vi "RT Main2.vi"() -> ()   [LabVIEW 2019]
uses:
  <vilib>/Platform/TimedLoop/XDataNode/timing_clust.ctl
  <vilib>/Platform/TimedLoop/XDataNode/nitl_modes.ctl
  <vilib>/Platform/TimedLoop/XDataNode/wakeup.ctl
  <vilib>/myRIO/Instrument Drivers/Onboard IO/AI/typedefs/AI Reference.ctl
  <vilib>/myRIO/Common/Instrument Driver Framework/Utilities/typedefs/myRIO Generic Hardware Reference.ctl
  <vilib>/myRIO/Common/Instrument Driver Framework/Utilities/typedefs/Hardware Version Enum.ctl
  <vilib>/myRIO/Common/Instrument Driver Framework/Utilities/typedefs/myRIO v1.0 Reference.ctl
  <vilib>/myRIO/Common/Instrument Driver Framework/Utilities/typedefs/Generic FPGA Reference.ctl
  <vilib>/myRIO/Common/Instrument Driver Framework/myRIO v1.0/AI/typedefs/AI Channels List.ctl
  <vilib>/myRIO/Common/Instrument Driver Framework/myRIO v1.0/AI/typedefs/AI Channels Enum.ctl
  <vilib>/myRIO/Common/Instrument Driver Framework/Utilities/typedefs/Analog Scaling Constants List.ctl
  <vilib>/myRIO/Common/Instrument Driver Framework/Utilities/typedefs/Analog Scaling Constants.ctl
  <vilib>/userDefined/High Color/nirio_resource_hc.ctl
  <vilib>/Simulation/Shared/_Datatypes/SIM SISO Transfer Function.ctl
  <vilib>/myRIO/Instrument Drivers/Onboard IO/AO/typedefs/AO Reference.ctl
  <vilib>/myRIO/Common/Instrument Driver Framework/myRIO v1.0/AO/typedefs/AO Channels List.ctl
  <vilib>/myRIO/Common/Instrument Driver Framework/myRIO v1.0/AO/typedefs/AO Channels Enum.ctl
  <vilib>/Analysis/Matrix/Datatypes/RealMatrix.ctl
  <vilib>/myRIO/Common/Instrument Driver Framework/Utilities/vis/Is FPGA Ref Available.vi
  <vilib>/myRIO/Common/Instrument Driver Framework/myRIO v1.0/AI/vis/myRIO v1.1 Open AI.vi
  <vilib>/myRIO/Instrument Drivers/Onboard IO/AI/vis/Read.vi
  <vilib>/Simulation/DiscreteLinear/Implementation/NILVSim Discrete Transfer Function Direct.llb/SIM Discrete Transfer Function Diagram (SISO).vi
  <vilib>/myRIO/Common/Instrument Driver Framework/myRIO v1.0/AO/vis/myRIO v1.1 Open AO.vi
  <vilib>/myRIO/Instrument Drivers/Onboard IO/AO/vis/Write.vi
  <vilib>/Analysis/7linalg.llb/Real Transpose Matrix.vi
  <vilib>/Analysis/baseanly.llb/Real A x B.vi
  <vilib>/myRIO/Common/Instrument Driver Framework/Utilities/vis/Validate Channels.vi
  <vilib>/myRIO/Common/Instrument Driver Framework/myRIO v1.0/AI/vis/myRIO v1.0 Reserve AI.vi
  <vilib>/Simulation/ContinuousLinear/Implementation/Shared/SIM Transfer Function Support.llb/SIM TransferFunction Normalize to Buffer.vi
  <vilib>/Simulation/DiscreteLinear/Implementation/Shared/SIM Init Discrete States.vi
  <vilib>/Simulation/DiscreteLinear/Implementation/NILVSim Discrete Transfer Function Direct.llb/SIM Transfer Function Direct core (SISO).vi
  <vilib>/myRIO/Common/Instrument Driver Framework/myRIO v1.0/AO/vis/myRIO v1.0 Reserve AO.vi
  <vilib>/myRIO/Common/Instrument Driver Framework/myRIO v1.0/AI/vis/myRIO v1.0 Build MUX Configuration AI.vi
  <vilib>/myRIO/Common/Instrument Driver Framework/myRIO v1.0/Resource Manager/vis/myRIO v1.0 Reserve Channel List.vi
  <vilib>/Simulation/ContinuousLinear/Implementation/Shared/SIM Transfer Function Support.llb/SIM TransferFunction Normalize.vi
  <vilib>/myRIO/Common/Instrument Driver Framework/myRIO v1.0/AO/vis/myRIO v1.0 Build MUX Configuration AO.vi
  <vilib>/myRIO/Common/Instrument Driver Framework/myRIO v1.0/Resource Manager/vis/myRIO v1.0 Reserve Channel.vi
  <vilib>/myRIO/Common/Instrument Driver Framework/myRIO v1.0/Resource Manager/vis/myRIO v1.0 Unreserve Channel.vi
  <vilib>/Simulation/Implementation/Shared/SIM Polynomials.llb/SIM Remove Zero Coefficients (DBL).vi
  <vilib>/myRIO/Common/Instrument Driver Framework/myRIO v1.0/Resource Manager/vis/myRIO v1.0 Build Mutex Name.vi
  <vilib>/Utility/VariantDataType/GetNumericInfo.vi
  <vilib>/Utility/error.llb/Error Cluster From Error Code.vi
  <vilib>/myRIO/Common/Instrument Driver Framework/myRIO v1.0/myRIO v1.1 Open.vi
  <vilib>/myRIO/Common/Instrument Driver Framework/myRIO v1.0/AI/vis/myRIO v1.0 Get Scaling Constants AI.vi
  <vilib>/myRIO/Common/Instrument Driver Framework/Utilities/vis/IO Manager.vi
  <vilib>/myRIO/Common/Instrument Driver Framework/Utilities/vis/Configuration Manager.vi
  <vilib>/myRIO/Common/Instrument Driver Framework/myRIO v1.0/myRIO v1.0 Close.vi
  <vilib>/myRIO/Common/Instrument Driver Framework/myRIO v1.0/AI/vis/myRIO v1.0 Read AI.vi
  <vilib>/Simulation/Implementation/Shared/SIM Polynomials.llb/SIM Divide Polynomials (DBL).vi
  <vilib>/Simulation/Implementation/Shared/SIM BuildSimErr.vi
  <vilib>/myRIO/Common/Instrument Driver Framework/myRIO v1.0/AO/vis/myRIO v1.0 Get Scaling Constants AO.vi
  <vilib>/myRIO/Common/Instrument Driver Framework/myRIO v1.0/AO/vis/myRIO v1.0 Write AO.vi
  <vilib>/Analysis/Matrix/Numeric/Conversions/Array To Matrix - RA.vi
  <vilib>/Analysis/Matrix/Numeric/Multiply/Multiply - R,RM.vi
  <vilib>/platform/TimedLoop/XDataNode/XDataNode.xnode
  <vilib>/myRIO/Express VI/Onboard IO/AI/AI Express VI.xnode
  <vilib>/myRIO/Instrument Drivers/Onboard IO/AI/vis/myRIO AI Open.xnode
  <vilib>/Simulation/Implementation/XNodeFramework/SimXNode/SimX.xnode
  <vilib>/myRIO/Express VI/Onboard IO/AO/AO Express VI.xnode
  <vilib>/myRIO/Instrument Drivers/Onboard IO/AO/vis/myRIO AO Open.xnode
  <vilib>/Platform/TimedLoop/XDataNode/XDNodeRunTimeDep.lvlib
  <vilib>/myRIO/Instrument Drivers/Onboard IO/AI/AI.lvlib
  <vilib>/myRIO/Instrument Drivers/Onboard IO/AO/AO.lvlib
  <vilib>/Analysis/Matrix/NI_Matrix.lvlib
  <vilib>/gmath/NI_Gmath.lvlib
  <vilib>/Analysis/NI_AALPro.lvlib
  <vilib>/Analysis/NI_AALBase.lvlib
panel:
  out "Control Law":string
  in  "Stop EM MLC":bool=TRUE
  out "x[um] 2":dbl(graph)
  out "u[A] 2":dbl(graph)
  out "iteration duration 2":i64(graph)
  in  "max J":dbl
  out "t MLC":dbl
  in  "MLC run time[s]":dbl
  out "J":dbl
  out "Wait For b":bool
  out "State":i16
  in  "PD run time[s]":dbl
  out "t [PD]":dbl
  in  "stop":bool
  in  "Kd":dbl
  in  "Kp":dbl
  out "iteration duration":i64(graph)
  out "u[A]":dbl(graph)
  out "x[um]":dbl(graph)
  in  "Stop EM PD":bool=TRUE
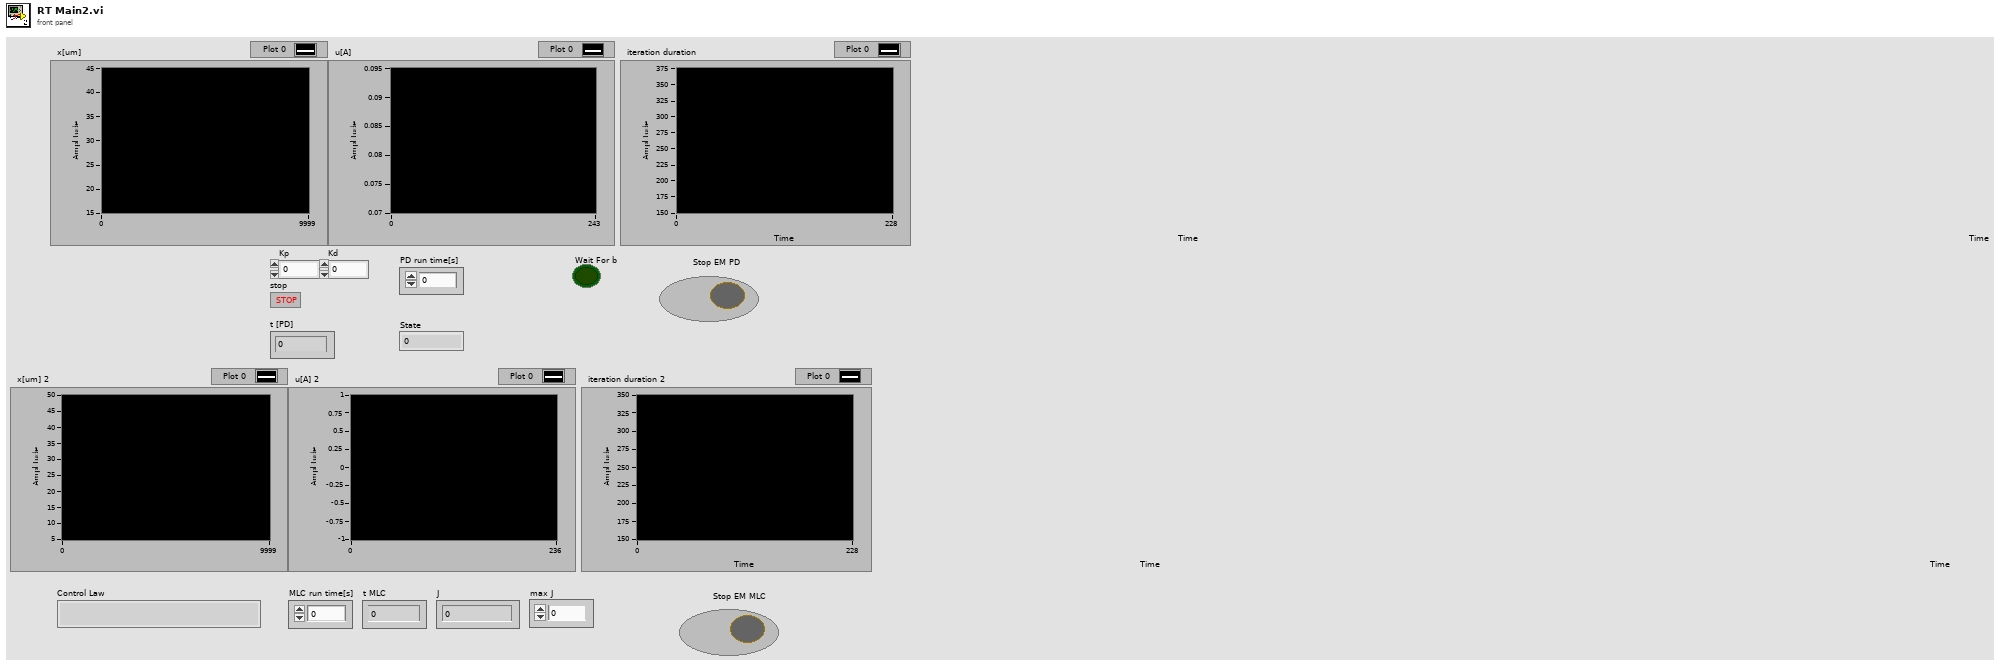
[diagram p1: front panel]
types:
  T1 = typedef "SIM SISO Transfer Function.ctl" = cluster{"Numerator":dbl[], "Denominator":dbl[]}
  T2 = typedef "AO.lvlib/AO Reference.ctl" = cluster{"myRIO Reference":T3, "AO Channel List":T7, "AO Scaling Constant List":T9}
  T3 = typedef "myRIO Generic Hardware Reference.ctl" = cluster{"myRIO Model":T4, "myRIO Hardware Reference":T5}
  T4 = typedef "Hardware Version Enum.ctl" = enum16{"Unknown", "myRIO-1900", "myRIO-1950", "roboRIO", "NI ELVIS RIO CM", "ELVIS III"}
  T5 = typedef "myRIO v1.0 Reference.ctl" = cluster{"Generic FPGA Reference":T6, "Allow multiple opens":bool}
  T6 = typedef "Generic FPGA Reference.ctl" = refnum<k20>
  T7 = typedef "AO Channels List.ctl" = T8[]
  T8 = typedef "AO Channels Enum.ctl" = enum16{"Not Connected", "AudioOut/Left", "AudioOut/Right", "C/AO0", "C/AO1", "A/AO0", "A/AO1", "B/AO0", "B/AO1"}
  T9 = typedef "Analog Scaling Constants List.ctl" = T10[]
  T10 = typedef "Analog Scaling Constants.ctl" = cluster{"LSB Weight (Volts)":dbl, "Offset (Volts)":dbl, "Signed?":bool}
  T11 = typedef "nirio_resource_hc.ctl" = tag
  T12 = typedef "AI.lvlib/AI Reference.ctl" = cluster{"myRIO Reference":T3, "AI Channels List":T13, "AI Scaling Constants List":T9}
  T13 = typedef "AI Channels List.ctl" = T14[]
  T14 = typedef "AI Channels Enum.ctl" = enum16{"Not Connected", "AudioIn/Left", "AudioIn/Right", "C/AI0", "C/AI1", "A/AI0", "A/AI1", "A/AI2", "A/AI3", "A/AI4", "A/AI5", "A/AI6", "A/AI7", "B/AI0", "B/AI1", "B/AI2", "B/AI3", "B/AI4", "B/AI5", "B/AI6", "B/AI7", "AI/AI0", "AI/AI1", "AI/AI2", "AI/AI3", "A/AI0 (DIFF)", "A/AI1 (DIFF)", "A/AI2 (DIFF)", "A/AI3 (DIFF)", "B/AI0 (DIFF)", "B/AI1 (DIFF)", "B/AI2 (DIFF)", "B/AI3 (DIFF)"}
  T15 = typedef "XDNodeRunTimeDep.lvlib/timing_clust.ctl" = cluster{"Expected End [f-1]":u64, "Actual End [f-1]":u64, "Finished Late? [f-1]":bool, "Expected End [i-1]":u64, "Actual End [i-1]":u64, "Finished Late? [i-1]":bool, "Expected Start [i]":u64, "Actual Start [i]":u64, "Expected Start [f]":u64, "Actual Start [f]":u64, "Source Name":string, "Structure Name":string, "Period":i64, "Deadline":i64, "Offset":i64, "Start":i64, "Priority":i32, "Timeout":i32, "Mode":T16, "Wakeup Reason":T17, "Error":errorcluster, "Source Type":string, "Secondary Source Type":string, "Global End Time":u64, "Global Start Time":u64, "Frame Duration":u64, "Iteration Duration":u64, "Assigned CPU":i32, "I/O Scan Engine Mode":u32}
  T16 = typedef "XDNodeRunTimeDep.lvlib/nitl_modes.ctl" = enum32{"No Change", "Process missed periods, maintain original phase", "Discard missed periods, maintain original phase", "Process missed periods, ignore original phase", "Discard missed periods, ignore original phase"}
  T17 = typedef "XDNodeRunTimeDep.lvlib/wakeup.ctl" = enum32{"Normal", "Aborted", "Asynchronous wakeup", "Timing source error", "Timed loop error", "Timeout"}
  T18 = enum16{"open", "replace", "create", "open or create", "replace or create", "replace or create with confirmation"}
  T19 = typedef "NI_Matrix.lvlib/RealMatrix.ctl" = dbl[][]
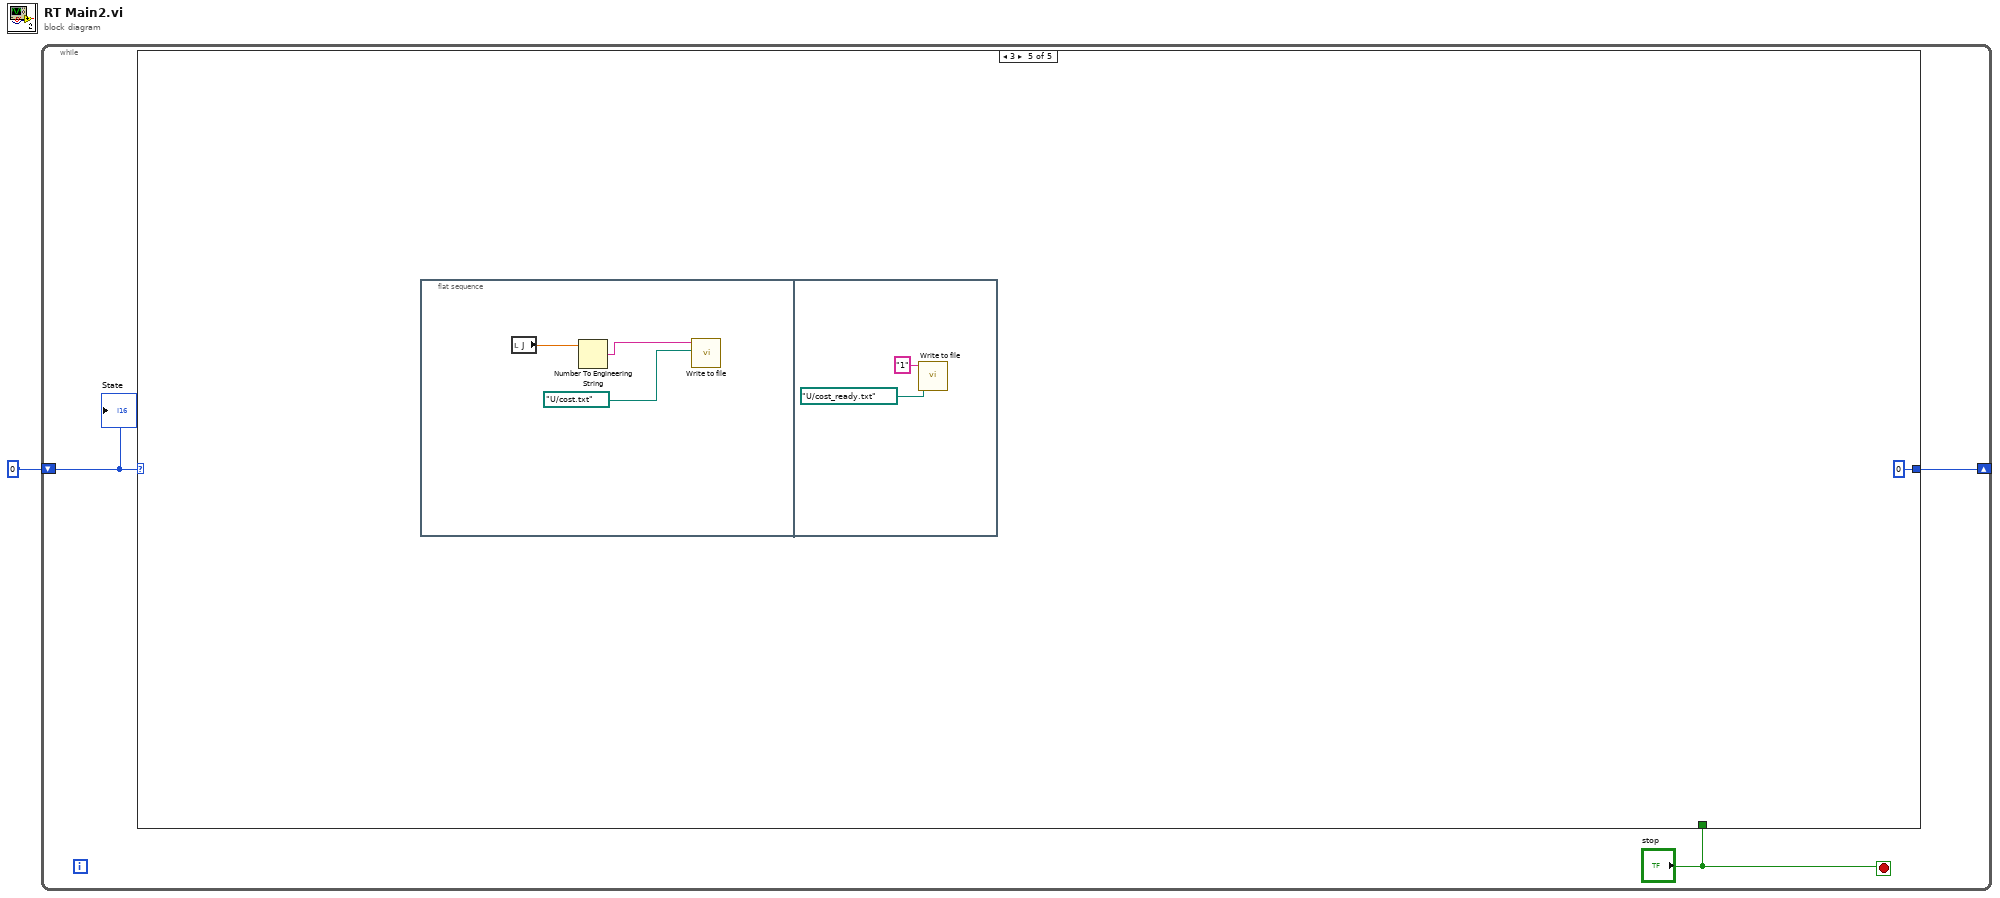
[diagram p0: block diagram]
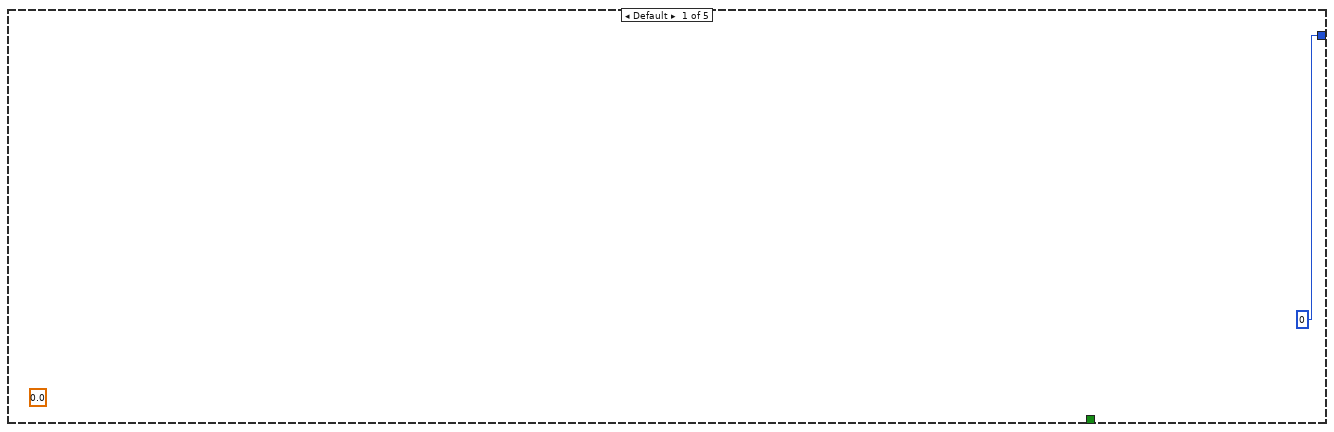
[diagram p2: hidden frame]
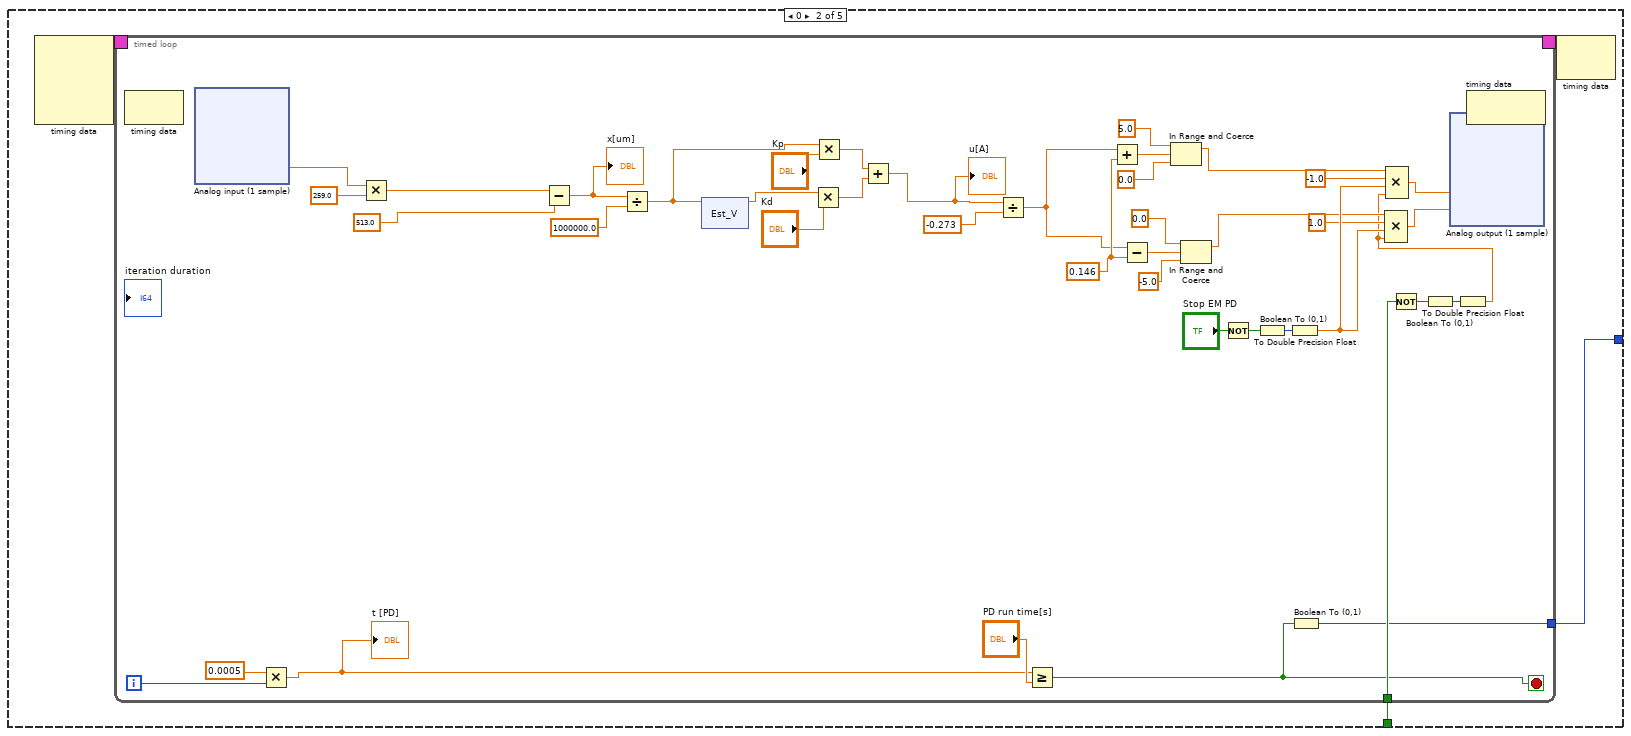
[diagram p3: hidden frame]
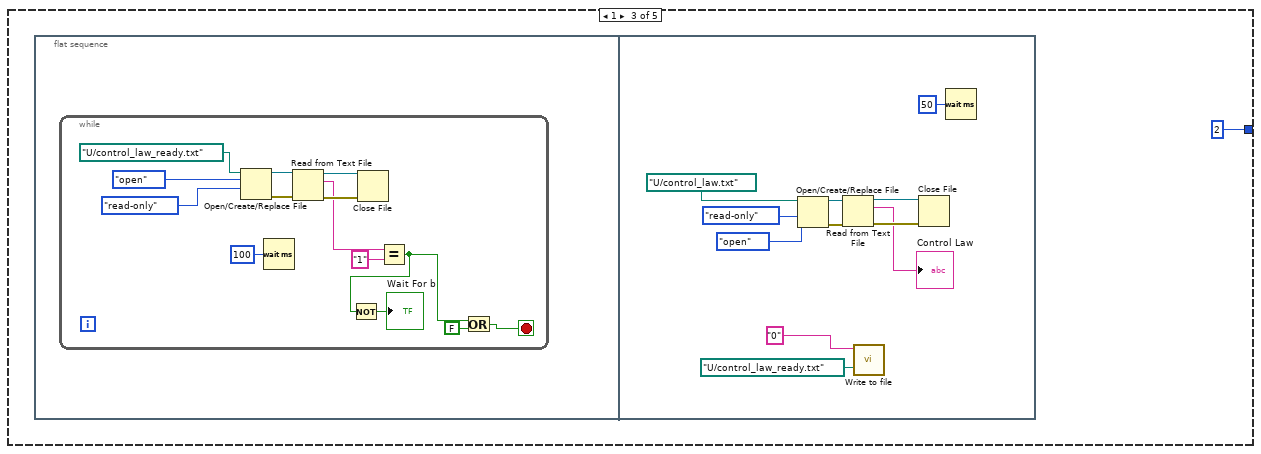
[diagram p4: hidden frame]
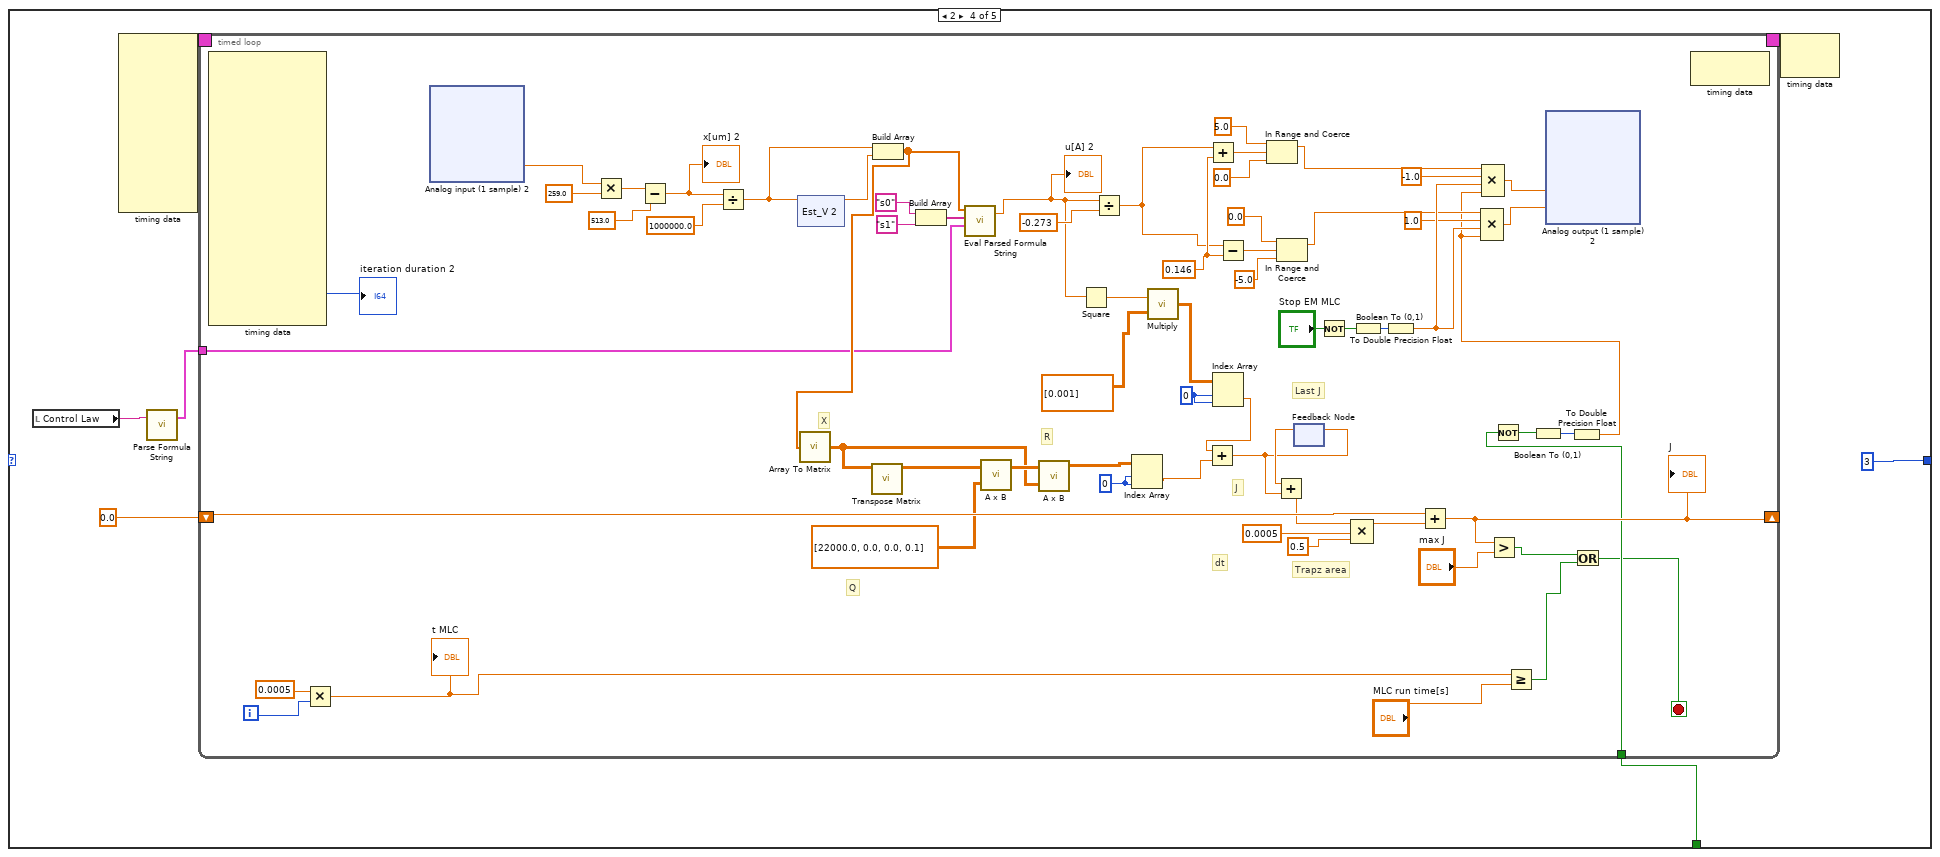
[diagram p5: hidden frame]
diagram:
  n1 = while {
    shift-right: [w3] -> _
    shift-left: i16 0 -> [w2]
    stop <- "stop" stop-if-true
    n2 = case shown="3" w2 {
      tunnel: "stop" -> [_ w7 _ w165 _]
      tunnel: [i16 0 w6 i16 2 i16 3 i16 0] -> w3
      frame Default {
        (unwired) 0.0
      }
      frame 0 {
        n3 = node-c288() -> (w9:T15)  [unwired: 4 in]
        n4 = timed-loop {
          timing: w9 -> [_]
          timing-out: [_] -> w8
          tunnel: w7 -> [w17]
          tunnel: [w11] -> w6
          i -> [w14]
          stop <- w12 stop-if-true
          w48 = 0.146 ("y")
          n5 = node-c288() -> ()  [unwired: 1 in, 1 out]
          n6 = xnode "Analog input (1 sample)"() -> ("C/AI1 (AI1)"=w36:dbl)  [unwired: 1 in, 1 out]
          n7 = Multiply(x=0.0005, y=w14) -> (x*y=w10:dbl)
          "t [PD]" <- w10
          n8 = Multiply(x=w36, y=259.0) -> (x*y=w35:dbl)
          n9 = Subtract(x=w35, y=513.0 ("x")) -> (x-y=w37:dbl)
          "x[um]" <- w37
          n10 = Divide(x=w37, y=1000000.0) -> (x/y=w24:dbl)
          n11 = xnode "Est_V"("input u(k)"=w24) -> ("output y(k)"=w23:dbl)  [unwired: 2 in, 1 out]
          n12 = Multiply(x=w23, y="Kd") -> (x*y=w25:dbl)
          n13 = Multiply(x=w24, y="Kp") -> (x*y=w26:dbl)
          n14 = Add(x=w26, y=w25) -> (x+y=w20:dbl)
          "u[A]" <- w20
          n15 = Divide(x=w20, y=-0.273) -> (x/y=w47:dbl)
          n16 = Greater Or Equal?(x=w10, y="PD run time[s]") -> (x >= y?=w12:bool)
          n17 = Add(x=w47, y=w48) -> (x+y=w46:dbl)
          n18 = Subtract(x=w47, y=w48) -> (x-y=w45:dbl)
          n19 = In Range and Coerce(upper limit=5.0, x=w46, lower limit=0.0) -> (coerced(x)=w33:dbl)  [unwired: 1 out]
          n20 = In Range and Coerce(upper limit=0.0, x=w45, lower limit=-5.0) -> (coerced(x)=w28:dbl)  [unwired: 1 out]
          n21 = Not(x="Stop EM PD") -> (.not. x?=w39:bool)
          n22 = Boolean To (0,1)(Boolean=w39) -> (0, 1=w38:i16)
          n23 = To Double Precision Float(number=w38) -> (double precision float=w30:dbl)
          n24 = Boolean To (0,1)(Boolean=w12) -> (0, 1=w11:i16)
          n25 = Not(x=w17) -> (.not. x?=w19:bool)
          n26 = Boolean To (0,1)(Boolean=w19) -> (0, 1=w18:i16)
          n27 = To Double Precision Float(number=w18) -> (double precision float=w16:dbl)
          n28 = Compound Arithmetic op=MULTIPLY(w28, 1.0 ("value"), w30, w16) -> (w27:dbl)
          n29 = Compound Arithmetic op=MULTIPLY(w33, -1.0 ("value"), w30, w16) -> (w31:dbl)
          n30 = xnode "Analog output (1 sample)"("C/AO0 (AO0)"=w31, "C/AO1 (AO1)"=w27) -> ()  [unwired: 1 in, 1 out]
          n31 = node-c288() -> ()  [unwired: 1 in, 1 out]
        }
        n32 = node-c288(w8) -> ()  [unwired: 1 out]
      }
      frame 1 {
        n33 = flat-sequence {
          frame #0 {
            n34 = while {
              stop <- w140 stop-if-true
              n35 = Open/Create/Replace File(file path (use dialog)=path "U:/control_law_ready.txt", operation (0:open)=T18."open", access (0:read/write)=enum16{"read/write", "read-only", "write-only"}."read-only") -> (refnum out=w147:refnum<file>, error out=w148:errorcluster)  [unwired: 3 in, 1 out]
              n36 = Wait (ms)(milliseconds to wait=u32 100) -> ()  [unwired: 1 out]
              n37 = Read from Text File(file (use dialog)=w147, error in=w148) -> (refnum out=w149:refnum<file>, text=w142:string, error out=w150:errorcluster)  [unwired: 2 in, 1 out]
              n38 = Close File(refnum=w149, error in=w150) -> ()  [unwired: 2 out]
              n39 = Equal?(x=w142, y="1") -> (x = y?=w139:bool)
              n40 = Not(x=w139) -> (.not. x?=→"Wait For b":bool)
              n41 = Or(x=w139, y=FALSE) -> (x .or. y?=w140:bool)
            }
          }
          frame #1 {
            n42 = Open/Create/Replace File(file path (use dialog)=path "U:/control_law.txt", operation (0:open)=T18."open", access (0:read/write)=enum16{"read/write", "read-only", "write-only"}."read-only") -> (refnum out=w161:refnum<file>, error out=w162:errorcluster)  [unwired: 3 in, 1 out]
            n43 = Read from Text File(file (use dialog)=w161, error in=w162) -> (refnum out=w156:refnum<file>, text=→"Control Law":string, error out=w157:errorcluster)  [unwired: 2 in, 1 out]
            n44 = call "Write to file.vi"("file path (use dialog)"=path "U:/control_law_ready.txt", "String"="0") -> ()  [unwired: 10 in]
            n45 = Close File(refnum=w156, error in=w157) -> ()  [unwired: 2 out]
            n46 = Wait (ms)(milliseconds to wait=u32 50) -> ()  [unwired: 1 out]
          }
        }
      }
      frame 2 {
        n47 = local read "Control Law"() -> (w167:string)
        n48 = node-c288() -> (w169:T15)  [unwired: 10 in]
        n49 = call <vilib>:"Parse Formula String.vi"("formula"=w167) -> ("Parsed Formula"=w166:cluster{"Table":i32[][], "Y Values":dbl[]})  [unwired: 1 in, 1 out]
        n50 = timed-loop {
          timing: w169 -> [_]
          timing-out: [_] -> w168
          shift-right: [w201] -> _
          shift-left: 0.0 -> [w203]
          tunnel: w166 -> [w202]
          tunnel: w165 -> [w177]
          i -> [w181]
          stop <- w174 stop-if-true
          w198 = 0 ("index (row)")
          w199 = 0 ("disabled index (col)")
          w229 = 0.146 ("y")
          # "R"
          # "Q"
          # "J"
          # "dt"
          # "Trapz area"
          # "Last J"
          # "X"
          n51 = node-c288() -> (→"iteration duration 2":i64)  [unwired: 1 in, 16 out]
          n52 = Multiply(x=0.0005, y=w181) -> (x*y=w176:dbl)
          "t MLC" <- w176
          n53 = xnode "Analog input (1 sample) 2"() -> ("C/AI1 (AI1)"=w217:dbl)  [unwired: 1 in, 1 out]
          n54 = Multiply(x=w217, y=259.0) -> (x*y=w216:dbl)
          n55 = Subtract(x=w216, y=513.0 ("x")) -> (x-y=w218:dbl)
          "x[um] 2" <- w218
          n56 = Divide(x=w218, y=1000000.0) -> (x/y=w180:dbl)
          n57 = xnode "Est_V 2"("input u(k)"=w180) -> ("output y(k)"=w179:dbl)  [unwired: 2 in, 1 out]
          n58 = Build Array(w180, w179) -> (w211:dbl[])
          n59 = call-poly <vilib>:"Array To Matrix.vi"("Real 1D Array"=w211) -> ("Real Matrix (Column Vector)"=w209:T19)
          n60 = call-poly <vilib>:"Transpose Matrix.vi"("Input Matrix"=w209) -> ("Matrix Transpose"=w213:T19)  [unwired: 9 in, 1 out]
          n61 = Build Array("s0", "s1") -> (w235:string[])
          n62 = call <vilib>:"Eval Parsed Formula String.vi"("Parsed Formula"=w202, "Variables"=w235, "X Values"=w211) -> ("y value"=w178:dbl)  [unwired: 1 in, 1 out]
          "u[A] 2" <- w178
          n63 = call-poly <vilib>:"A x B.vi"("B"=T19 [[22000.0, 0.0], [0.0, 0.1]], "A"=w213) -> ("A x B"=w212:T19)  [unwired: 1 out]
          n64 = call-poly <vilib>:"A x B.vi"("B"=w209, "A"=w212) -> ("A x B"=w205:T19)  [unwired: 1 out]
          n65 = Square(x=w178) -> (x^2=w210:dbl)
          n66 = Divide(x=w178, y=-0.273) -> (x/y=w228:dbl)
          n67 = Index Array(array=w205, index (row)=w198, index (col)=w198) -> (element=w204:dbl)
          n68 = call-poly <vilib>:"Multiply.vi"("Real Matrix A"=T19 [[0.001]], "Real Scalar c"=w210) -> ("c * A"=w207:T19)
          n69 = Add(x=w228, y=w229) -> (x+y=w227:dbl)
          n70 = Index Array(array=w207, index (row)=w199, index (col)=w199) -> (element=w206:dbl)
          n71 = Add ("Add.vi")(x=w206, y=w204) -> (x+y=w183:dbl)
          n72 = Subtract(x=w228, y=w229) -> (x-y=w226:dbl)
          n73 = In Range and Coerce(upper limit=5.0, x=w227, lower limit=0.0) -> (coerced(x)=w195:dbl)  [unwired: 1 out]
          n74 = In Range and Coerce(upper limit=0.0, x=w226, lower limit=-5.0) -> (coerced(x)=w190:dbl)  [unwired: 1 out]
          n75 = feedback-in #1(w183) -> ()
          n76 = feedback #1() -> (w208:dbl)  [unwired: 1 in]
          n77 = Add ("Add.vi")(x=w208, y=w183) -> (x+y=w187:dbl)
          n78 = Not(x="Stop EM MLC") -> (.not. x?=w220:bool)
          n79 = Compound Arithmetic op=MULTIPLY(w187, 0.0005 ("y"), 0.5 ("value")) -> (w184:dbl)
          n80 = Boolean To (0,1)(Boolean=w220) -> (0, 1=w219:i16)
          n81 = To Double Precision Float(number=w219) -> (double precision float=w192:dbl)
          n82 = Add ("Add.vi")(x=w203, y=w184) -> (x+y=w201:dbl)
          "J" <- w201
          n83 = Greater?(x=w201, y="max J") -> (0:w170:bool)
          n84 = Not(x=w177) -> (.not. x?=w197:bool)
          n85 = Greater Or Equal?(x=w176, y="MLC run time[s]") -> (x >= y?=w175:bool)
          n86 = Boolean To (0,1)(Boolean=w197) -> (0, 1=w196:i16)
          n87 = To Double Precision Float(number=w196) -> (double precision float=w189:dbl)
          n88 = Compound Arithmetic op=MULTIPLY(w190, 1.0 ("value"), w192, w189) -> (w188:dbl)
          n89 = Compound Arithmetic op=MULTIPLY(w195, -1.0 ("value"), w192, w189) -> (w193:dbl)
          n90 = xnode "Analog output (1 sample) 2"("C/AO0 (AO0)"=w193, "C/AO1 (AO1)"=w188) -> ()  [unwired: 1 in, 1 out]
          n91 = Or(x=w170, y=w175) -> (x .or. y?=w174:bool)
          n92 = node-c288() -> ()  [unwired: 1 in, 1 out]
        }
        n93 = node-c288(w168) -> ()  [unwired: 1 out]
      }
      frame 3 {
        n94 = flat-sequence {
          frame #0 {
            n95 = local read "J"() -> (w325:dbl)
            n96 = Number To Engineering String(4:w325) -> (0:w324:string)  [unwired: 3 in]
            n97 = call "Write to file.vi"("file path (use dialog)"=path "U:/cost.txt", "String"=w324) -> ()  [unwired: 10 in]
          }
          frame #1 {
            n98 = call "Write to file.vi"("file path (use dialog)"=path "U:/cost_ready.txt", "String"="1") -> ()  [unwired: 10 in]
          }
        }
      }
    }
    "State" <- w2
  }
